vi "Backlash (DBL Array).vi"(1 "reinitialize? (F)":bool, 2 "initial value":dbl[](array[numeric]) format="%.2f", 3 "deadband":dbl[](array[numeric]) format="%.2f", 4 "input":dbl[](array[numeric]) format="%.2f") -> (0 "output":dbl[](array[numeric]) format="%.2f")   [LabVIEW 2020, in "NI_AdvCtrl_nonlinear.lvlib"]
doc: "LabVIEW no longer supports this VI. You can obtain similar functionality by installing the LabVIEW Simulation Module.\n\nImplements a backlash or deadband function. Output will not change until the input value differs from the current output by at least the deadband amount."
uses:
  <vilib>/addons/control/advanced/NI_AdvCtrl_nonlinear.lvlib
  <vilib>/addons/control/pid/NI_PID_pid.lvlib
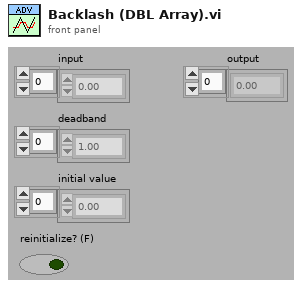
[diagram p1: front panel]
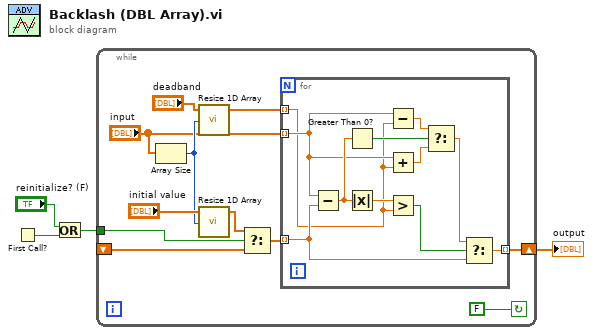
[diagram p0: block diagram]
diagram:
  n1 = First Call?() -> (First Call?: T/F=w4:bool)
  n2 = Or(x="reinitialize? (F)", y=w4) -> (x .or. y?=w2:bool)
  n3 = while {
    tunnel: w2 -> [w12]
    shift-left: _ -> [w13]
    shift-right: [w15] -> w1
    stop <- FALSE continue-if-true
    n4 = Array Size(array="input") -> (size(s)=w8:i32)
    n5 = call <vilib>:"Resize 1D Array.vi"("array size"=w8, "input array"="deadband") -> ("output array"=w6:dbl[])  [unwired: 3 out]
    n6 = call <vilib>:"Resize 1D Array.vi"("array size"=w8, "input array"="initial value") -> ("output array"=w10:dbl[])  [unwired: 3 out]
    n7 = Select(t=w10, s=w12, f=w13) -> (s? t:f=w14:dbl[])
    n8 = for {
      tunnel: [w24] -> w15 mode=indexing
      tunnel: w14 -> [w18] mode=indexing
      tunnel: "input" -> [w17] mode=indexing
      tunnel: w6 -> [w16] mode=indexing
      n9 = Subtract(x=w17, y=w18) -> (x-y=w23:dbl)
      n10 = Greater Than 0?(x=w23) -> (x > 0?=w22:bool)
      n11 = Absolute Value(x=w23) -> (abs(x)=w26:dbl)
      n12 = Subtract(x=w17, y=w16) -> (x-y=w20:dbl)
      n13 = Add(x=w17, y=w16) -> (x+y=w21:dbl)
      n14 = Greater?(x=w26, y=w16) -> (0:w25:bool)
      n15 = Select(t=w20, s=w22, f=w21) -> (s? t:f=w19:dbl)
      n16 = Select(t=w19, s=w25, f=w18) -> (s? t:f=w24:dbl)
    }
  }
  "output" <- w1
